vi "Filtering - per-appender threshold.vi"(8 "error in (no error)":errorcluster) -> (0 "error out":errorcluster)   [LabVIEW 2026, in "Tests.lvlib"]
doc: "Integration test. Verifies that a single Log call fans out to every registered appender: registers three queue-mode relay appenders, logs one Info message, and asserts each appender's queue receives exactly one Statement with identical payload. Every gate except fan-out is held open (global threshold at floor, permissive filters, unbounded queues), so a missing element can only be a fan-out defect.\n\nImplements LMBR-T-030 -> SRS-019, SRS-028. Assert-level IDs: Test-ID-Assert-Checklist.md."
uses:
  Tests.lvlib
  src/TypeDefs/Severity.ctl
  <vilib>/addons/_JKI Toolkits/Caraya/classes/Assert/Assert Equal Value_Variant.vi
  <vilib>/addons/_JKI Toolkits/Caraya/classes/Assert/Assert True.vi
  <vilib>/addons/_JKI Toolkits/Caraya/classes/Test/Test.lvclass
  src/Lumberjack.lvlib
  src/Public/Logger.lvclass/Logger.lvclass
  <vilib>/addons/_JKI Toolkits/Caraya/classes/Assert/Assert.lvclass
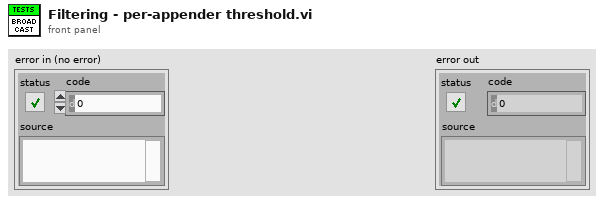
[diagram p1: front panel]
types:
  T1 = typedef "Lumberjack.lvlib/Severity.ctl" = enum16{"OFF", "FATAL", "ERROR", "WARN", "INFO", "DEBUG", "TRACE", "ALL"}
  T2 = typedef "Lumberjack.lvlib/Statement.ctl" = cluster{"timestamp":timestamp, "level":T1, "sourceTag":string, "originVI":string, "message":string}
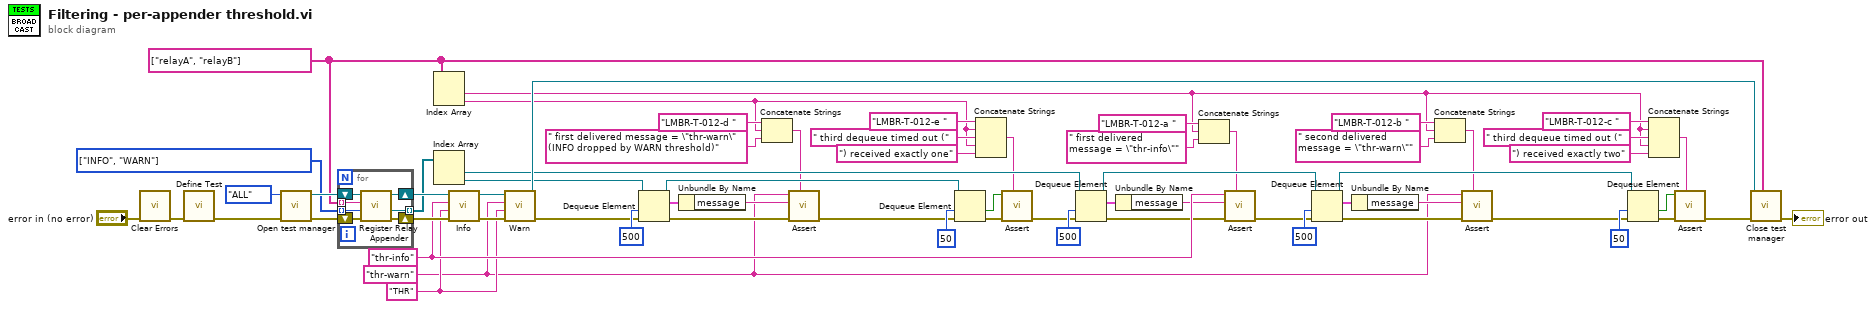
[diagram p0: block diagram]
diagram:
  w5 = "thr-warn" ("message")
  w57 = T1[] [enum."INFO", enum."WARN"] items=["OFF", "FATAL", "ERROR", "WARN", "INFO", "DEBUG", "TRACE", "ALL"]
  w53 = "THR" ("sourceTag")
  w3 = string[] ["relayA", "relayB"]
  w59 = "thr-info" ("message")
  n1 = call <vilib>:"Clear Errors.vi"("error in (no error)"="error in (no error)") -> ("error out"=w1:errorcluster)  [unwired: 5 in, 1 out]
  n2 = call <vilib>:"Define Test.vi"("error in (no error)"=w1) -> ("error out"=w66:errorcluster)  [unwired: 9 in, 1 out]
  n3 = call "Open test manager.vi"("error in (no error)"=w66, "globalThreshold"=Severity."ALL") -> ("error out"=w62:errorcluster, "Logger out"=w63:refnum<class "Logger.lvclass">)  [unwired: 8 in]
  n4 = for {
    shift-right: [w71] -> w61
    shift-left: w63 -> [w73]
    shift-right: [w70] -> w60
    shift-left: w62 -> [w72]
    tunnel: w3 -> [w69] mode=indexing
    tunnel: [w68] -> w52 mode=indexing
    tunnel: w57 -> [w67] mode=indexing
    n5 = call "Register Relay Appender.vi"("error in (no error)"=w72, "threshold"=w67, "id in"=w69, "Logger in"=w73) -> ("error out"=w70:errorcluster, "relayQueue"=w68:refnum<queue>, "Logger out"=w71:refnum<class "Logger.lvclass">)  [unwired: 4 in, 1 out]
  }
  n6 = Index Array(array=w3) -> (element #1=w27:string, element #2=w4:string)  [unwired: 2 in]
  n7 = Index Array(array=w52) -> (element #1=w45:refnum<queue>, element #2=w6:refnum<queue>)  [unwired: 2 in]
  n8 = call "Info.vi"("error in (no error)"=w60, "sourceTag"=w53, "message"=w59, "Logger in"=w61) -> ("error out"=w55:errorcluster, "Logger out"=w56:refnum<class "Logger.lvclass">)  [unwired: 6 in]
  n9 = call "Warn.vi"("error in (no error)"=w55, "sourceTag"=w53, "message"=w5, "Logger in"=w56) -> ("error out"=w8:errorcluster, "Logger out"=w54:refnum<class "Logger.lvclass">)  [unwired: 6 in]
  n10 = Dequeue Element(queue=w6, timeout in ms (-1)=500, error in (no error)=w8) -> (queue out=w17:refnum<queue>, element=w20:T2, error out=w18:errorcluster)  [unwired: 1 out]
  n11 = Unbundle By Name(w20) -> ("message"=w19:string)
  n12 = Concatenate Strings("LMBR-T-012-d ", w4, " first delivered message = \"thr-warn\" (INFO dropped by WARN threshold)") -> (w9:string)
  n13 = call-poly <vilib>:"Assert.vi"("Label"=w9, "error in (no error)"=w18, "Actual"=w19, "Expected"=w5) -> ("error out"=w16:errorcluster)  [unwired: 6 in, 1 out]
  n14 = Dequeue Element(queue=w17, timeout in ms (-1)=50, error in (no error)=w16) -> (timed out?=w22:bool, error out=w23:errorcluster)  [unwired: 2 out]
  n15 = Concatenate Strings("LMBR-T-012-e ", w4, " third dequeue timed out (", w4, ") received exactly one") -> (w10:string)
  n16 = call-poly <vilib>:"Assert.vi"("Label"=w10, "error in (no error)"=w23, "True?"=w22) -> ("error out"=w7:errorcluster)  [unwired: 7 in, 1 out]
  n17 = Dequeue Element(queue=w45, timeout in ms (-1)=500, error in (no error)=w7) -> (queue out=w38:refnum<queue>, element=w50:T2, error out=w44:errorcluster)  [unwired: 1 out]
  n18 = Unbundle By Name(w50) -> ("message"=w49:string)
  n19 = Concatenate Strings("LMBR-T-012-a ", w27, " first delivered message = \"thr-info\"") -> (w26:string)
  n20 = call-poly <vilib>:"Assert.vi"("Label"=w26, "error in (no error)"=w44, "Actual"=w49, "Expected"=w59) -> ("error out"=w39:errorcluster)  [unwired: 6 in, 1 out]
  n21 = Dequeue Element(queue=w38, timeout in ms (-1)=500, error in (no error)=w39) -> (queue out=w37:refnum<queue>, element=w42:T2, error out=w40:errorcluster)  [unwired: 1 out]
  n22 = Unbundle By Name(w42) -> ("message"=w41:string)
  n23 = Concatenate Strings("LMBR-T-012-b ", w27, " second delivered message = \"thr-warn\"") -> (w25:string)
  n24 = call-poly <vilib>:"Assert.vi"("Label"=w25, "error in (no error)"=w40, "Actual"=w41, "Expected"=w5) -> ("error out"=w36:errorcluster)  [unwired: 6 in, 1 out]
  n25 = Dequeue Element(queue=w37, timeout in ms (-1)=50, error in (no error)=w36) -> (timed out?=w46:bool, error out=w47:errorcluster)  [unwired: 2 out]
  n26 = Concatenate Strings("LMBR-T-012-c ", w27, " third dequeue timed out (", w27, ") received exactly two") -> (w28:string)
  n27 = call-poly <vilib>:"Assert.vi"("Label"=w28, "error in (no error)"=w47, "True?"=w46) -> ("error out"=w58:errorcluster)  [unwired: 7 in, 1 out]
  n28 = call "Close test manager.vi"("queueIDList"=w3, "error in (no error)"=w58, "Logger in"=w54) -> ("error out"=→"error out":errorcluster)  [unwired: 6 in]
